vi "AddMessageToLog.vi"(8 "error in (no error)":errorcluster, 10 "Message":T2, 11 "AppContextIn":T1) -> (0 "error out":errorcluster, 3 "AppContextOut":T1)   [LabVIEW 2011]
uses:
  030 - EVENTS/03 - ToMessageHandlerProcess/ToMessageHandlerEvent.ctl
  030 - EVENTS/03 - ToMessageHandlerProcess/enumMessageCriticity.ctl
  MessageHandlerContext.ctl
  050 - CONFIG/00 - ApplicationConfig/Ctrls/EnumFgvConfigCommand.ctl
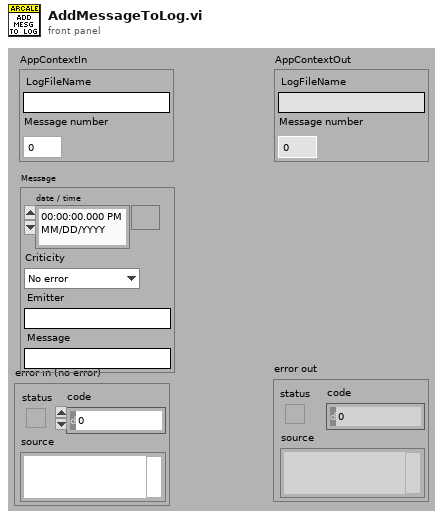
[diagram p1: front panel]
types:
  T1 = typedef "MessageHandlerContext.ctl" = cluster{"LogFileName":string, "Message number":i32}
  T2 = typedef "ToMessageHandlerEvent.ctl" = cluster{"date / time":timestamp, "Criticity":T3, "Emitter":string, "Message":string}
  T3 = typedef "enumMessageCriticity.ctl" = enum16{"No error", "Info", "Warning", "Error", "Fatal error"}
  T4 = typedef "EnumFgvConfigCommand.ctl" = enum16{"Load", "Get", "Set", "Save To Disk"}
  T5 = typedef "ApplicationConfig.ctl" = cluster{"Data Path":path, "MessageHandlerConfig":T6, "Simulation":bool, "Dictionnary":string}
  T6 = typedef "MessageHandlerConfig.ctl" = cluster{"Max log files":u32, "Max messages per file":u32}
  T7 = typedef "ApplicationPaths.ctl" = cluster{"Data Path":path, "Log Path":path, "Tmp Path":path}
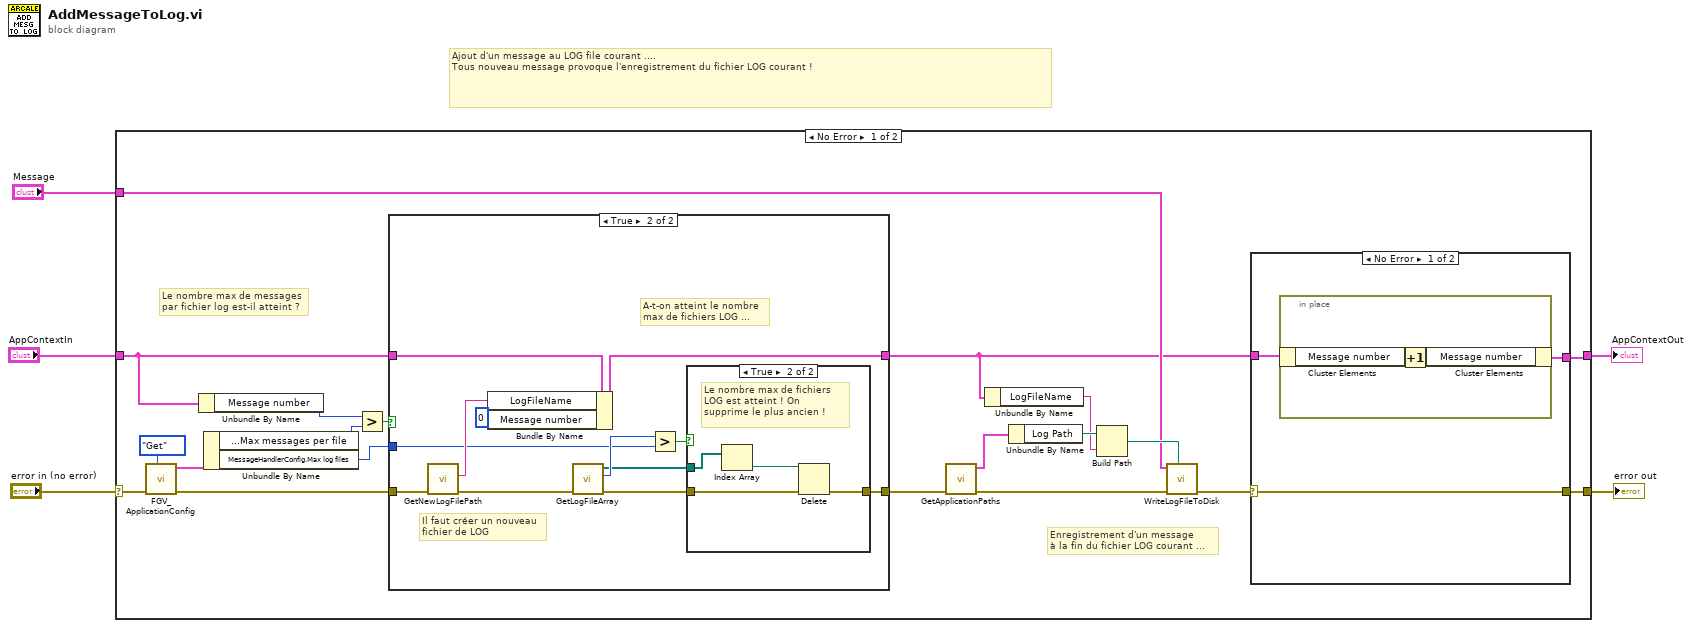
[diagram p0: block diagram]
diagram:
  # "Ajout d'un message au LOG file courant ....\nTous nouveau message provoque l'enregistrement du fichier LOG courant !"
  n1 = case shown="No Error" "error in (no error)" {
    selector: "error in (no error)" -> [w25 w53]
    tunnel: [w9 w53] -> w4
    tunnel: "AppContextIn" -> [w19 w52]
    tunnel: [w8 w52] -> w2
    tunnel: "Message" -> [w11 _]
    frame No Error {
      # "Enregistrement d'un message\nà la fin du fichier LOG courant ..."
      # "Le nombre max de messages\npar fichier log est-il atteint ?"
      n2 = call "FGV_ApplicationConfig.vi"("Command"=EnumFgvConfigCommand."Get", "error in (no error)"=w25) -> ("error out"=w21:errorcluster, "ApplicationConfigOut"=w23:T5)  [unwired: 8 in]
      n3 = Unbundle By Name(w19) -> ("Message number"=w12:i32)
      n4 = Unbundle By Name(w23) -> ("MessageHandlerConfig.Max messages per file"=w22:u32, "MessageHandlerConfig.Max log files"=w13:u32)
      n5 = Greater?(x=w12, y=w22) -> (0:w20:bool)
      n6 = case shown="True" w20 {
        tunnel: w21 -> [w33 w46]
        tunnel: w19 -> [w34 w45]
        tunnel: [w34 w43] -> w6
        tunnel: [w33 w36] -> w17
        tunnel: w13 -> [_ w40]
        frame False {
          # "Le nombre max de messages\npar fichier n'est pas encore\natteint !"
        }
        frame True {
          # "A-t-on atteint le nombre\nmax de fichiers LOG ..."
          # "Il faut créer un nouveau\nfichier de LOG"
          n7 = call "GetNewLogFilePath.vi"("error in (no error)"=w46) -> ("error out"=w42:errorcluster, "New log filename"=w44:string)  [unwired: 8 in, 1 out]
          n8 = Bundle By Name(cluster=w45, "LogFileName"=w44, "Message number"=0) -> (w43:T1)
          n9 = call "GetLogFileArray.vi"("error in (no error)"=w42) -> ("error out"=w38:errorcluster, "LogFileNumber"=w41:u32, "LogFileArray"=w37:path[])  [unwired: 8 in]
          n10 = Greater?(x=w41, y=w40) -> (0:w39:bool)
          n11 = case shown="True" w39 {
            tunnel: w38 -> [w47 w50]
            tunnel: w37 -> [_ w51]
            tunnel: [w47 w49] -> w36
            frame False {
              # "Le nombre max de fichiers\nn'est pas atteint !"
            }
            frame True {
              # "Le nombre max de fichiers\nLOG est atteint ! On \nsupprime le plus ancien !"
              n12 = Index Array(array=w51) -> (element=w48:path)  [unwired: 1 in]
              n13 = Delete(path (use dialog)=w48, error in=w50) -> (error out=w49:errorcluster)  [unwired: 3 in, 2 out]
            }
          }
        }
      }
      n14 = call "GetApplicationPaths.vi"("error in (no error)"=w17) -> ("error out"=w18:errorcluster, "ApplicationPath"=w16:T7)  [unwired: 9 in]
      n15 = Unbundle By Name(w6) -> ("LogFileName"=w7:string)
      n16 = Unbundle By Name(w16) -> ("Log Path"=w15:path)
      n17 = Build Path(base path=w15, name or relative path=w7) -> (appended path=w14:path)
      n18 = call "WriteLogFileToDisk.vi"("Log File path"=w14, "error in (no error)"=w18, "Message"=w11) -> ("error out"=w10:errorcluster)  [unwired: 8 in]
      n19 = case shown="No Error" w10 {
        selector: w10 -> [w28 w31]
        tunnel: w6 -> [w27 w32]
        tunnel: [w28 w31] -> w9
        tunnel: [w26 w32] -> w8
        frame No Error {
          n20 = in-place {
            n21 = in-place-cluster #1(w27) -> ("Message number"=w30:i32)
            n22 = Increment(x=w30) -> (x+1=w29:i32)
            n23 = in-place-cluster #1("Message number"=w29) -> (w26:T1)
          }
        }
        frame Error {
        }
      }
    }
    frame Error {
    }
  }
  "error out" <- w4
  "AppContextOut" <- w2
